vi "KillAllConnections.vi"(8 "error in (no error)":errorcluster, 11 "TcpServer in":refnum<class "TcpServer.lvclass">) -> (0 "error out":errorcluster, 3 "TcpServer out":refnum<class "TcpServer.lvclass">)   [LabVIEW 2022 SP3, in "TcpServer.lvlib" / "TcpServer.lvclass"]
uses:
  TcpServer.lvclass
  C:/Users/jakub/repos/gh/sw4sys/lv-tcp-server-sample/LoggingActor/Source/LoggingActor/LoggingActor/LoggingActor.lvclass
  LoggingActor/Source/LoggingActor/LoggingActor/LoggingActor.lvclass/LoggingActor.ctl
  TcpServer.lvclass/TcpServer.ctl
  <vilib>/ActorFramework/Message Enqueuer/Message Enqueuer.lvclass/Message Enqueuer.ctl
  LoggingActor/Source/LoggingActor/LoggingActor/Read Logger.vi
  <vilib>/ActorFramework/Message Enqueuer/Enqueue.vi
  Connection/Connection Messages/Kill Msg/Kill Msg.lvclass
  C:/Program Files (x86)/National Instruments/LabVIEW 2022/vi.lib/ActorFramework/Message/Message.lvclass
  <vilib>/ActorFramework/Message Priority Queue/Priority Enqueue.vi
  Logger/Source/Logger/Logger.lvclass
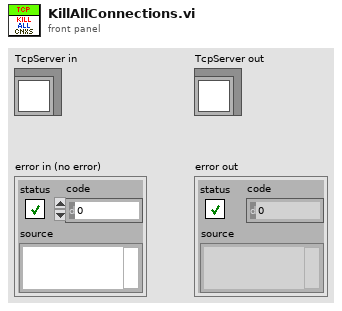
[diagram p1: front panel]
types:
  T1 = map{u64, refnum<class "Message Enqueuer.lvclass">}
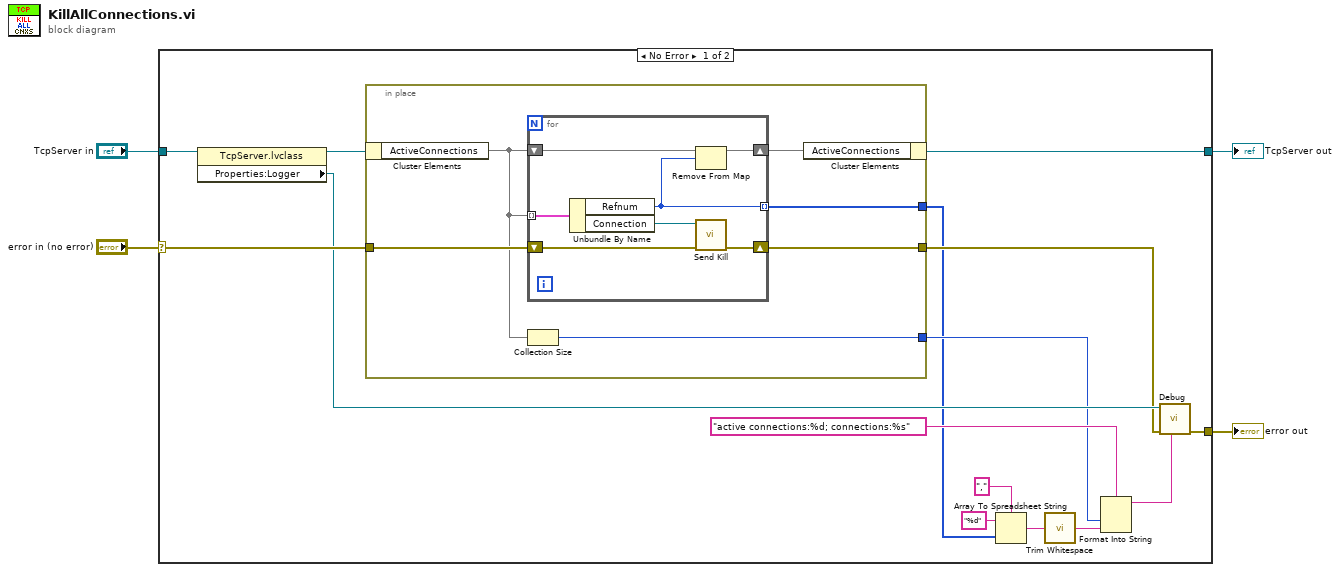
[diagram p0: block diagram]
diagram:
  n1 = case shown="No Error" "error in (no error)" {
    selector: "error in (no error)" -> [w17 w34]
    tunnel: [w13 w34] -> w3
    tunnel: [w18 w33] -> w1
    tunnel: "TcpServer in" -> [w19 w33]
    frame No Error {
      n2 = property class="TcpServer.lvclass"(reference=w19) -> (reference out=w16:refnum<class "TcpServer.lvclass">, "Properties:Logger"=w15:refnum<class "Logger.lvclass">)  [unwired: 1 in, 1 out]
      n3 = in-place {
        in-place-border: w17 -> [w25]
        in-place-border: [w24] -> w14
        in-place-border: [w21] -> w7
        in-place-border: [w20] -> w8
        n4 = in-place-cluster #1(w16) -> ("ActiveConnections"=w22:T1)
        n5 = for {
          tunnel: w22 -> [w32] mode=indexing
          shift-right: [w29] -> w24
          shift-left: w25 -> [w30]
          shift-right: [w27] -> w23
          shift-left: w22 -> [w28]
          tunnel: [w26] -> w21 mode=indexing
          n6 = Unbundle By Name(w32) -> ("Refnum"=w26:u64, "Connection"=w31:refnum<class "Message Enqueuer.lvclass">)
          n7 = Remove From Map(10:w26, 11:w28) -> (3:w27:T1)  [unwired: 2 out]
          n8 = call "Send Kill.vi"("error in (no error)"=w30, "Message Enqueuer"=w31) -> ("error out"=w29:errorcluster)  [unwired: 8 in, 1 out]
        }
        n9 = Collection Size(1:w22) -> (0:w20:i32)
        n10 = in-place-cluster #1("ActiveConnections"=w23) -> (w18:refnum<class "TcpServer.lvclass">)
      }
      n11 = Array To Spreadsheet String(delimiter (Tab)=",", array=w7, 3:"%d" ("format string")) -> (spreadsheet string=w9:string)
      n12 = call <vilib>:"Trim Whitespace.vi"("string"=w9) -> ("trimmed string"=w5:string)  [unwired: 1 in]
      n13 = Format Into String(format string="active connections:%d; connections:%s", w8, w5) -> (resulting string=w6:string)  [unwired: 2 in, 1 out]
      n14 = call-dynamic "Debug.vi"("Message"=w6, "error in (no error)"=w14, "Logger in"=w15) -> ("error out"=w13:errorcluster)  [unwired: 5 in, 1 out]
    }
    frame Error {
    }
  }
  "error out" <- w3
  "TcpServer out" <- w1
